vi "Log Data.vi"(0 "Test Inputs":T2 {"Duration of the pulse in s" format="%#.5g"; "Input Voltage Vin1 in V" format="%#.5g"}, 1 "Save Scope Data?":bool, 5 "Test Results":T1 {"Second Edge - Settling Time in s" format="%#.5p"; "First Edge - Settling Time in s" format="%#.5p"; "Actual Sample Rate" format="%#.5g"}, 7 "DataLogger File Path":path, 11 "error in (no error)":errorcluster) -> (15 "error out":errorcluster)   [LabVIEW 2020, in "LDO Line Transient.lvlib"]
uses:
  LDO Line Transient.lvlib
  Typedefs/Test Inputs.ctl
  Typedefs/Settling Time Calc Option.ctl
  Typedefs/Advance Settings.ctl
  Typedefs/Adv Settings Setup Instr.ctl
  Reusables/Instrument APIs/Load Output Function.ctl
  Typedefs/Test Results.ctl
  <vilib>/Utility/file.llb/Write Delimited Spreadsheet (string).vi
panel:
  # "Load SMU"
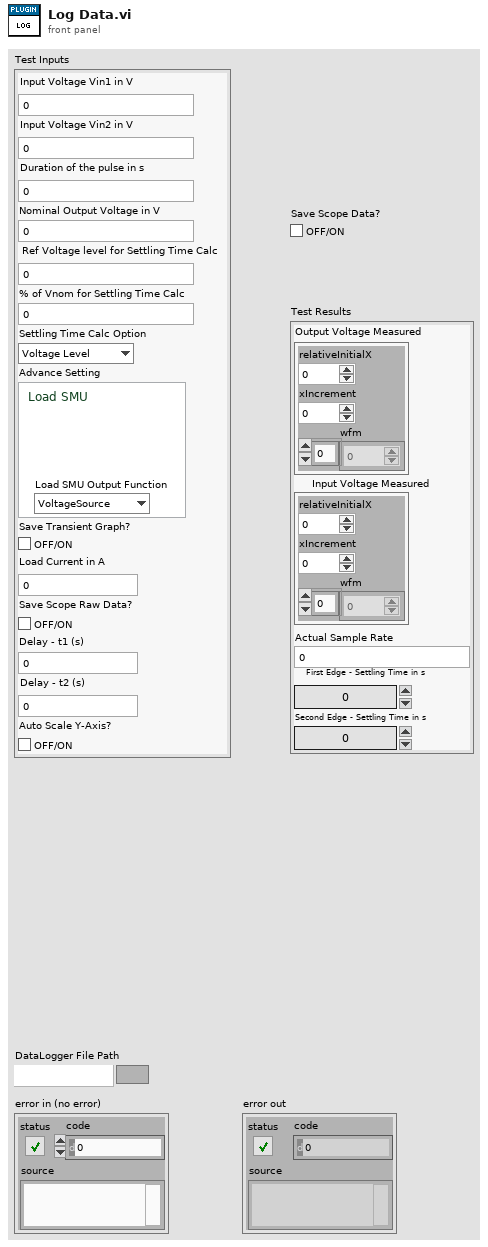
[diagram p1: front panel]
types:
  T1 = typedef "LDO Line Transient.lvlib/Test Results.ctl" = cluster{"Output Voltage Measured":cluster{"relativeInitialX":dbl, "xIncrement":dbl, "wfm":dbl[]}, "Input Voltage Measured":cluster{"relativeInitialX":dbl, "xIncrement":dbl, "wfm":dbl[]}, "Actual Sample Rate":dbl, "First Edge - Settling Time in s":dbl, "Second Edge - Settling Time in s":dbl}
  T2 = typedef "LDO Line Transient.lvlib/Test Inputs.ctl" = cluster{"Input Voltage Vin1 in V":dbl, "Input Voltage Vin2 in V":dbl, "Duration of the pulse in s":dbl, "Nominal Output Voltage in V":dbl, "Ref Voltage level for Settling Time Calc":dbl, "% of Vnom for Settling Time Calc":dbl, "Settling Time Calc Option":T3, "Advance Setting":T4, "Save Transient Graph?":bool, "Load Current in A":dbl, "Save Scope Raw Data?":bool, "Delay - t1 (s)":dbl, "Delay - t2 (s)":dbl, "Auto Scale Y-Axis?":bool}
  T3 = typedef "LDO Line Transient.lvlib/Settling Time Calc Option.ctl" = enum16{"Voltage Level ", "Percentage of Vnom"}
  T4 = typedef "LDO Line Transient.lvlib/Advance Settings.ctl" = cluster{"Prepare":T5}
  T5 = typedef "LDO Line Transient.lvlib/Adv Settings Setup Instr.ctl" = cluster{"Load SMU Output Function":T6}
  T6 = typedef "Load Output Function.ctl" = enum16{"VoltageSource", "CurrentSource"}
  T7 = enum16{"open", "replace", "create", "open or create", "replace or create", "replace or create with confirmation"}
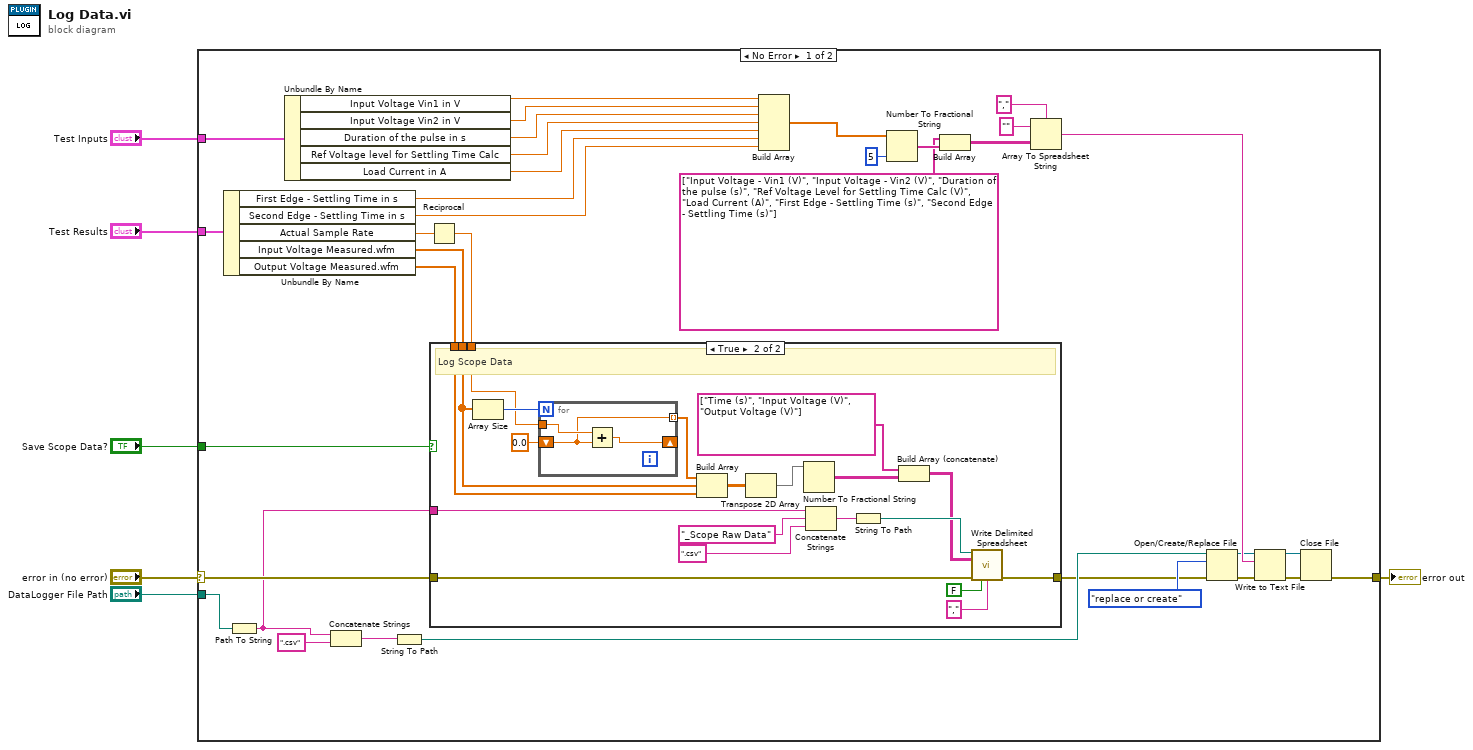
[diagram p0: block diagram]
diagram:
  n1 = case shown="No Error" "error in (no error)" {
    selector: "error in (no error)" -> [w15 w66]
    tunnel: [w37 w66] -> w5
    tunnel: "Test Inputs" -> [w41 _]
    tunnel: "Test Results" -> [w40 _]
    tunnel: "DataLogger File Path" -> [w16 _]
    tunnel: "Save Scope Data?" -> [w8 _]
    frame No Error {
      n2 = Unbundle By Name(w40) -> ("First Edge - Settling Time in s"=w38:dbl, "Second Edge - Settling Time in s"=w7:dbl, "Actual Sample Rate"=w12:dbl, "Input Voltage Measured.wfm"=w10:dbl[], "Output Voltage Measured.wfm"=w9:dbl[])
      n3 = Path To String(path=w16) -> (string=w13:string)
      n4 = Unbundle By Name(w41) -> ("Input Voltage Vin1 in V"=w33:dbl, "Input Voltage Vin2 in V"=w39:dbl, "Duration of the pulse in s"=w23:dbl, "Ref Voltage level for Settling Time Calc"=w21:dbl, "Load Current in A"=w20:dbl)
      n5 = Concatenate Strings(w13, ".csv" ("format string")) -> (w25:string)
      n6 = String To Path(string=w25) -> (path=w24:path)
      n7 = Reciprocal(x=w12) -> (1/x=w11:dbl)
      n8 = case shown="True" w8 {
        tunnel: w15 -> [w42 w62]
        tunnel: [w42 w61] -> w14
        tunnel: w13 -> [_ w58]
        tunnel: w11 -> [_ w54]
        tunnel: w10 -> [_ w51]
        tunnel: w9 -> [_ w50]
        frame False {
          # "Skip Scope Log File"
        }
        frame True {
          # "Log Scope Data"
          n9 = Array Size(array=w51) -> (size(s)=w55:i32)
          n10 = for {
            N: w55 -> [_]
            tunnel: w54 -> [w64]
            shift-right: [w65] -> _
            shift-left: 0.0 -> [w63]
            tunnel: [w63] -> w52 mode=indexing
            n11 = Add(x=w64, y=w63) -> (x+y=w65:dbl)
          }
          n12 = Build Array(w52, w51, w50) -> (w49:dbl[][])
          n13 = Transpose 2D Array(2D array=w49) -> (transposed array=w46:dbl[][])
          n14 = Number To Fractional String(number=w46) -> (F-format string=w45:string[][])  [unwired: 3 in]
          n15 = Concatenate Strings(w58, "_Scope Raw Data" ("string"), ".csv" ("format string")) -> (w59:string)
          n16 = String To Path(string=w59) -> (path=w56:path)
          n17 = Build Array (concatenate)(string[] ["Time (s)", "Input Voltage (V)", "Output Voltage (V)"], w45) -> (w44:string[][])
          n18 = call-poly <vilib>:"Write Delimited Spreadsheet.vi"("file path (dialog if empty)"=w56, "2D data"=w44, "error in (no error)"=w62, "transpose? (no:F)"=FALSE, "delimiter (\\t)"="," ("delimiter (\\t)")) -> ("error out"=w61:errorcluster)  [unwired: 9 in, 1 out]
        }
      }
      n19 = Build Array(w33, w39, w23, w21, w20, w38, w7) -> (w22:dbl[])
      n20 = Number To Fractional String(number=w22, precision (6)=i16 5) -> (F-format string=w19:string[])  [unwired: 2 in]
      n21 = Build Array(string[] ["Input Voltage - Vin1 (V)", "Input Voltage - Vin2 (V)", "Duration of the pulse (s)", "Ref Voltage Level for Settling Time Calc (V)", "Load Current (A)", "First Edge - Settling Time (s)", "Second Edge - Settling Time (s)"] ("new element/subarray"), w19) -> (w17:string[][])
      n22 = Array To Spreadsheet String(delimiter (Tab)=",", array=w17, 3:"" ("format string")) -> (spreadsheet string=w34:string)
      n23 = Open/Create/Replace File(file path (use dialog)=w24, error in=w14, operation (0:open)=T7."replace or create") -> (refnum out=w29:refnum<file>, error out=w31:errorcluster)  [unwired: 3 in, 1 out]
      n24 = Write to Text File(file (use dialog)=w29, text=w34, error in=w31) -> (refnum out=w28:refnum<file>, error out=w30:errorcluster)  [unwired: 1 in, 1 out]
      n25 = Close File(refnum=w28, error in=w30) -> (error out=w37:errorcluster)  [unwired: 1 out]
    }
    frame Error {
    }
  }
  "error out" <- w5
